vi "Base Command Gen.vi"(7 "Query":bool, 8 "nn2+":dbl[](array[numeric]), 9 "nn1":dbl=nan, 10 "Command":string, 11 "xx":i32=-1) -> (3 "Command":string)   [LabVIEW 2019]
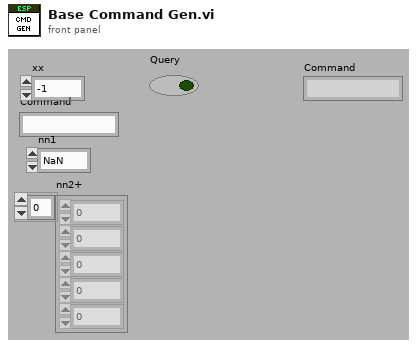
[diagram p1: front panel]
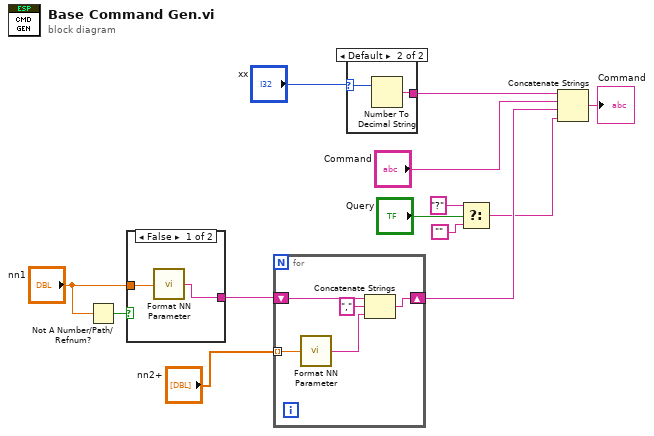
[diagram p0: block diagram]
diagram:
  n1 = Not A Number/Path/Refnum?(number/path/refnum="nn1") -> (NaN/Path/Refnum?=w12:bool)
  n2 = case shown="False" w12 {
    tunnel: "nn1" -> [w15 _]
    tunnel: [w14 _] -> w10
    frame False {
      n3 = call "Format NN Parameter.vi"("nn1"=w15) -> ("String"=w14:string)
    }
    frame True {
    }
  }
  n4 = for {
    shift-right: [w18] -> w6
    shift-left: w10 -> [w20]
    tunnel: "nn2+" -> [w17] mode=indexing
    n5 = call "Format NN Parameter.vi"("nn1"=w17) -> ("String"=w16:string)
    n6 = Concatenate Strings(w20, "," ("string"), w16) -> (w18:string)
  }
  n7 = case shown="Default" "xx" {
    selector: "xx" -> [_ w22]
    tunnel: [_ w21] -> w8
    frame -1 {
    }
    frame Default {
      n8 = Number To Decimal String(number=w22) -> (decimal integer string=w21:string)  [unwired: 1 in]
    }
  }
  n9 = Select(t="?", s="Query", f="") -> (s? t:f=w2:string)
  n10 = Concatenate Strings(w8, "Command", w6, w2) -> (→"Command":string)
